vi "AirHeaterModel.vi"(1 "Tenv":dbl, 2 "Ts":dbl, 3 "u":dbl, 4 "Tout":dbl) -> (0 "Tout":dbl)   [LabVIEW 2023]
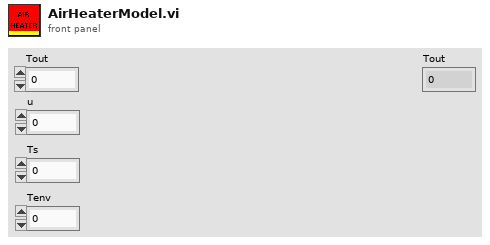
[diagram p1: front panel]
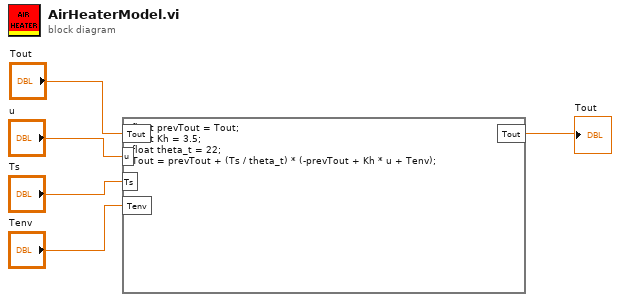
[diagram p0: block diagram]
diagram:
  n1 = formula code="float prevTout = Tout;\nfloat Kh = 3.5;\nfloat theta_t = 22;\nTout = prevTout + (Ts / theta_t) * (-prevTout + Kh * u + Tenv);"("Tout"="Tout", "u"="u", "Ts"="Ts", "Tenv"="Tenv") -> ("Tout"=→"Tout":dbl)
